vi "AddAxisExtendedDataConfiguration.vi"(6 "argument":i32, 8 "error in (no error)":errorcluster, 9 "axis extended data signal":u32(ring)=10 items=["AmplifierPeakCurrent"=303, "AmplifierTemperature"=309, "AnalogInput0"=10, "AnalogInput1"=11, "AnalogInput2"=28, "AnalogInput3"=29, "AnalogOutput0"=36, "AnalogOutput1"=37, "AnalogOutput2"=38, "AnalogOutput3"=39, "AnalogSensorInput"=446, "BoardRevision"=407, "BusVoltage"=375, "BusVoltageNegative"=441, "CapacitanceSensorRawPosition"=415, "CommandOutputType"=389, "ControlEffort"=282, "CurrentCommand"=8, "CurrentFeedback"=7, "DataAcquisitionSamples"=234, "DriveFeedforwardOutput"=404, "DriveMemoryDouble"=42, "DriveMemoryDoublePointer"=206, "DriveMemoryFloat"=41, "DriveMemoryFloatPointer"=205, "DriveMemoryInt16"=157, "DriveMemoryInt16Pointer"=203, "DriveMemoryInt32"=40, "DriveMemoryInt32Pointer"=202, "DriveMemoryInt8"=158, "DriveMemoryInt8Pointer"=204, "DriveTimer"=44, "DriveTimerMax"=319, "DriveTypeID"=305, "EncoderCosine"=27, "EncoderSine"=26, "EnDatAbsolutePosition"=269, "EthernetDebuggingInformation"=365, "FaultPositionFeedback"=372, "FirmwareRevision"=408, "FirmwareVersionBuild"=318, "FirmwareVersionMajor"=315, "FirmwareVersionMinor"=316, "FirmwareVersionPatch"=317, "FPGAVersion"=304, "GalvoLaserOutput"=409, "GalvoLaserPowerCorrectionOutput"=414, "InternalErrorCode"=314, "IOBoardInstalled"=374, "LastTickCounter"=405, "LatchedMarkerPosition"=331, "LoopTransmissionAfter"=31, "LoopTransmissionBefore"=30, "MarkerSearchDistance"=320, "MaximumVoltage"=388, "ModbusBitMasterInputBits"=290, "ModbusBitMasterOutputBits"=291, "ModbusRegDoubleMasterInputWords"=298, "ModbusRegDoubleMasterOutputWords"=299, "ModbusRegInt16MasterInputWords"=292, "ModbusRegInt16MasterOutputWords"=293, "ModbusRegInt32MasterInputWords"=294, "ModbusRegInt32MasterOutputWords"=295, "ModbusRegSingleMasterInputWords"=296, "ModbusRegSingleMasterOutputWords"=297, "MotorCommutationAngle"=373, "MotorTemperature"=447, "MXAbsolutePosition"=311, "NpaqSyncoutStatus"=366, "PhaseACurrentFeedback"=24, "PhaseAVoltageCommand"=300, "PhaseBCurrentFeedback"=25, "PhaseBVoltageCommand"=301, "PhaseCVoltageCommand"=302, "PiezoVoltageCommand"=376, "PiezoVoltageFeedback"=377, "PositionCalibrationGalvo"=419, "PositionCommandDrive"=98, "PositionCommandGalvo"=237, "PositionDetectorVoltage"=235, "PositionFeedbackDrive"=88, "PositionFeedbackGalvo"=327, "ProcessorTemperature"=442, "PSOBitArrayIndex"=310, "PSOCounter1"=229, "PSOCounter2"=230, "PSOCounter3"=231, "PSODistanceArrayIndex"=308, "PSOStatus"=43, "PSOWindow1"=232, "PSOWindow1ArrayIndex"=306, "PSOWindow2"=233, "PSOWindow2ArrayIndex"=307, "ResoluteAbsolutePosition"=369, "ResoluteStatus"=449, "ResolverChannel1"=267, "ResolverChannel2"=268, "ServoUpdateRate"=312, "SettlingTime"=313, "STOStatus"=443, "TemperatureSensor"=332, "TimeSinceReset"=387, "ZHSDifference"=32, "ZHSFiltered"=35, "ZHSSum"=33, "ZHSUnfiltered"=34], 10 "axisExtendedIndex in":i32, 11 "controller in":refnum<k24>) -> (0 "error out":errorcluster, 2 "axisExtendedIndex out":i32, 3 "controller out":refnum<k24>)   [LabVIEW 2010]
uses:
  c:/aerotech/controller/stable/a3200/pc/labview/2010/bin/Aerotech.A3200.dll
  bin/Aerotech.A3200.dll
  c:/aerotech/controller/stable/a3200/pc/labview/2010/bin/Aerotech.A3200.LabVIEW.dll
  bin/Aerotech.A3200.LabVIEW.dll
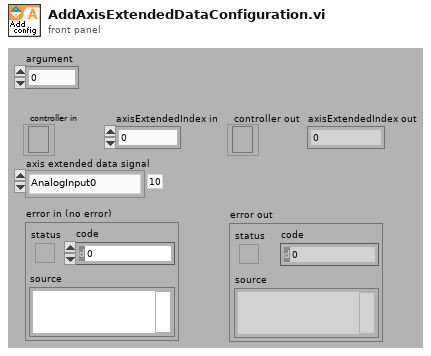
[diagram p1: front panel]
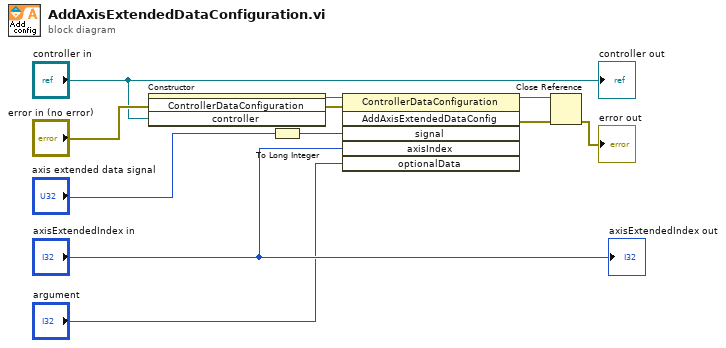
[diagram p0: block diagram]
diagram:
  n1 = constructor class="ControllerDataConfiguration"(error in="error in (no error)", "controller"="controller in") -> (reference out=w10:refnum<k24>, error out=w9:errorcluster)  [unwired: 2 in, 2 out]
  n2 = To Long Integer(number="axis extended data signal") -> (32bit integer=w3:i32)
  n3 = invoke class="ControllerDataConfiguration" method="AddAxisExtendedDataConfig"(reference=w10, error in=w9, "signal"=w3, "axisIndex"="axisExtendedIndex in", "optionalData"="argument") -> (reference out=w6:refnum<k24>, error out=w5:errorcluster)  [unwired: 1 in, 4 out]
  n4 = Close Reference(reference=w6, error in (no error)=w5) -> (error out=→"error out":errorcluster)
  "controller out" <- "controller in"
  "axisExtendedIndex out" <- "axisExtendedIndex in"
